vi "Data Preparation.vi"(5 "Data":T1) -> (2 "Measured Data Out":dbl[](array[numeric]))   [LabVIEW 2018]
uses:
  Controls/DataType.ctl
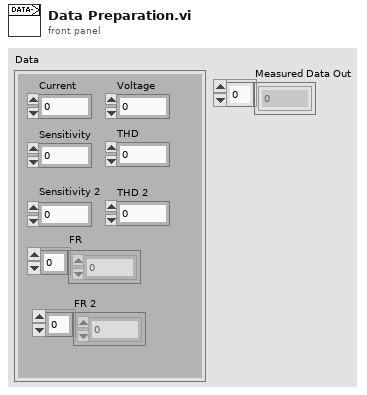
[diagram p1: front panel]
types:
  T1 = typedef "DataType.ctl" = cluster{"Current":dbl, "Voltage":dbl, "Sensitivity":dbl, "THD":dbl, "FR":dbl[], "Sensitivity 2":dbl, "THD 2":dbl, "FR 2":dbl[]}
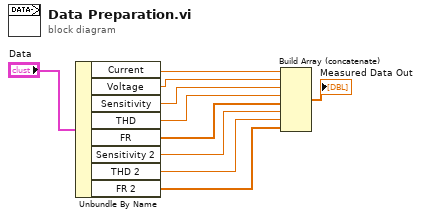
[diagram p0: block diagram]
diagram:
  n1 = Unbundle By Name("Data") -> ("Current"=w8:dbl, "Voltage"=w7:dbl, "Sensitivity"=w6:dbl, "THD"=w4:dbl, "FR"=w5:dbl[], "Sensitivity 2"=w3:dbl, "THD 2"=w2:dbl, "FR 2"=w1:dbl[])
  n2 = Build Array (concatenate)(w8, w7, w6, w4, w5, w3, w2, w1) -> (→"Measured Data Out":dbl[])
